vi "Swerve Drive.vi"(0 "X":dbl, 1 "Rot. Point X":dbl, 3 "Rot. Point Y":dbl, 5 "Y":dbl, 7 "Z":dbl, 11 "Error In":errorcluster, 12 "Robot Centric?":bool=TRUE, 13 "Autonomous?":bool, 14 "Yaw":dbl) -> (4 "Front Left Output":dbl, 6 "Front Right Output":dbl, 8 "Back Left Output":dbl, 10 "Back Right Output":dbl, 15 "Error Out":errorcluster)   [LabVIEW 2017]
uses:
  Public/Documents/Cross The Road Electronics/Phoenix-LabVIEW/Motor Controller/Controls/CTRE_Phoenix_MotorControl_ControlMode.ctl
  <vilib>/Rock Robotics/Network Tables/NT Read Number.vi
  <vilib>/Rock Robotics/Network Tables/NT Write Numeric Array.vi
panel:
  in  "Robot Length":dbl=33.5
  in  "Robot Width":dbl=28.5
  # "Swerve Drive Teleoperated Control\nFRC Team 34"
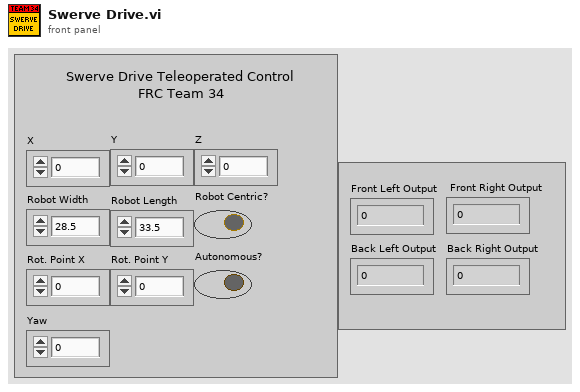
[diagram p1: front panel]
types:
  T1 = enum16{"Front Left", "Front Right", "Back Left", "Back Right"}
  T2 = typedef "CTRE_Phoenix_MotorControl_ControlMode.ctl" = u16
  T3 = typedef "WPI_MotorControlDeviceRef.ctl" = cluster{"DeviceStatus":errorcluster, "Type":T4, "PWM":cluster{"PWM Channel":T5, "DeadBand":T6}, "CAN":cluster{"Device Number":u8, "SetOutput VI Ref":variant, "GetOutput VI Ref":variant, "Enable VI Ref":variant, "Disable VI Ref":variant, "Data":variant}, "Invert":bool, "DIO PWM":cluster{"PWM \"Enable\" Channel":T5, "DIOChannel":T7, "PWM Rate":dbl}}
  T4 = typedef "WPI_MotorControlType.ctl" = enum16{"PWM", "CAN", "DIO PWM"}
  T5 = typedef "FPGA_DIOPWMChannel.ctl" = enum8{"PWM 0", "PWM 1", "PWM 2", "PWM 3", "PWM 4", "PWM 5", "PWM 6", "PWM 7", "PWM 8", "PWM 9", "PWM MXP 0", "PWM MXP 1", "PWM MXP 2", "PWM MXP 3", "PWM MXP 4", "PWM MXP 5", "PWM MXP 6", "PWM MXP 7", "PWM MXP 8", "PWM MXP 9", "Invalid"}
  T6 = typedef "WPI_PWMDeadband.ctl" = cluster{"Name":string, "maxPositivePwm":i32, "minPositivePwm":i32, "centerPwm":i32, "maxNegativePwm":i32, "minNegativePwm":i32, "angularRange":u16}
  T7 = typedef "FPGA_DIOChannel.ctl" = enum8{"DIO 0", "DIO 1", "DIO 2", "DIO 3", "DIO 4", "DIO 5", "DIO 6", "DIO 7", "DIO 8", "DIO 9", "DIO MXP 0", "DIO MXP 1", "DIO MXP 2", "DIO MXP 3", "DIO MXP 4", "DIO MXP 5", "DIO MXP 6", "DIO MXP 7", "DIO MXP 8", "DIO MXP 9", "DIO MXP 10", "DIO MXP 11", "DIO MXP 12", "DIO MXP 13", "DIO MXP 14", "DIO MXP 15", "SPI Port CS1", "SPI Port CS2", "SPI Port CS3", "SPI Port MISO", "SPI Port MOSI", "Invalid"}
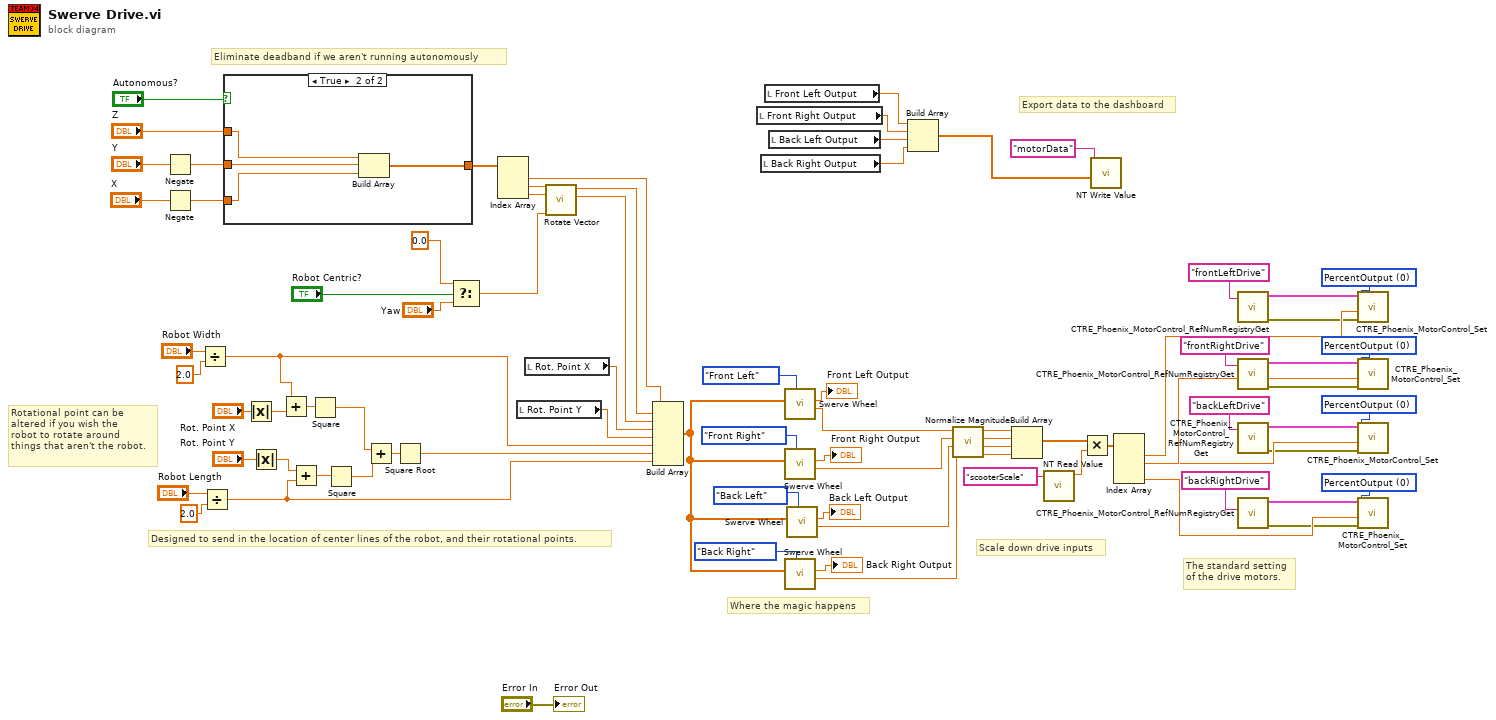
[diagram p0: block diagram]
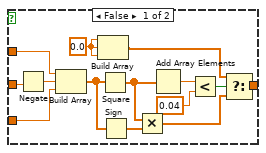
[diagram p2: hidden frame]
diagram:
  w12 = T2 0 items=["PercentOutput"=0, "Position"=1, "Velocity"=2, "Current"=3, "Follower"=5, "MotionProfile"=6, "MotionMagic"=7, "MotionMagicArc"=8, "MotionProfileArc"=10, "Disabled"=15] ("Control Mode")
  w13 = T2 0 items=["PercentOutput"=0, "Position"=1, "Velocity"=2, "Current"=3, "Follower"=5, "MotionProfile"=6, "MotionMagic"=7, "MotionMagicArc"=8, "MotionProfileArc"=10, "Disabled"=15] ("Control Mode")
  w14 = T2 0 items=["PercentOutput"=0, "Position"=1, "Velocity"=2, "Current"=3, "Follower"=5, "MotionProfile"=6, "MotionMagic"=7, "MotionMagicArc"=8, "MotionProfileArc"=10, "Disabled"=15] ("Control Mode")
  w15 = T2 0 items=["PercentOutput"=0, "Position"=1, "Velocity"=2, "Current"=3, "Follower"=5, "MotionProfile"=6, "MotionMagic"=7, "MotionMagicArc"=8, "MotionProfileArc"=10, "Disabled"=15] ("Control Mode")
  # "Export data to the dashboard"
  # "Rotational point can be \naltered if you wish the \nrobot to rotate around \nthings that aren't the robot."
  # "Scale down drive inputs"
  # "Eliminate deadband if we aren't running autonomously"
  # "Where the magic happens"
  # "The standard setting\nof the drive motors."
  # "Designed to send in the location of center lines of the robot, and their rotational points."
  n1 = Negate(x="Y") -> (-x=w33:dbl)
  n2 = Negate(x="X") -> (-x=w32:dbl)
  n3 = Divide(x="Robot Width", y=2.0) -> (x/y=w55:dbl)
  n4 = Divide(x="Robot Length", y=2.0) -> (x/y=w53:dbl)
  n5 = case shown="True" "Autonomous?" {
    tunnel: w33 -> [w86 w99]
    tunnel: [w85 w97] -> w81
    tunnel: "Z" -> [w84 w100]
    tunnel: w32 -> [w83 w98]
    frame False {
      w92 = 0.0 ("element")
      n6 = Negate(x=w86) -> (-x=w88:dbl)
      n7 = Build Array(w84, w88, w83) -> (w91:dbl[])
      n8 = Build Array(w92, w92, w92) -> (w93:dbl[])
      n9 = Square(x=w91) -> (x^2=w89:dbl[])
      n10 = Sign(1:w91) -> (0:w90:dbl[])
      n11 = Multiply(x=w89, y=w90) -> (x*y=w87:dbl[])
      n12 = Add Array Elements(numeric array=w89) -> (sum=w96:dbl)
      n13 = Less?(x=w96, y=0.04 ("x")) -> (x < y?=w94:bool)
      n14 = Select(t=w93, s=w94, f=w87) -> (s? t:f=w85:dbl[])
    }
    frame True {
      n15 = Build Array(w100, w99, w98) -> (w97:dbl[])
    }
  }
  n16 = Absolute Value(x="Rot. Point X") -> (abs(x)=w67:dbl)
  n17 = Absolute Value(x="Rot. Point Y") -> (abs(x)=w64:dbl)
  n18 = Add(x=w55, y=w67) -> (x+y=w66:dbl)
  n19 = Add(x=w64, y=w53) -> (x+y=w65:dbl)
  n20 = Square(x=w66) -> (x^2=w62:dbl)
  n21 = Square(x=w65) -> (x^2=w63:dbl)
  n22 = Add(x=w62, y=w63) -> (x+y=w61:dbl)
  n23 = Square Root(x=w61) -> (sqrt(x)=w54:dbl)
  n24 = Select(t=0.0, s="Robot Centric?", f="Yaw") -> (s? t:f=w74:dbl)
  n25 = Index Array(array=w81) -> (element #1=w60:dbl, element #2=w76:dbl, element #3=w75:dbl)  [unwired: 3 in]
  n26 = local read "Rot. Point Y"() -> (w56:dbl)
  n27 = local read "Rot. Point X"() -> (w57:dbl)
  n28 = call "Rotate Vector.vi"("Angle"=w74, "X"=w75, "Y"=w76) -> ("X'"=w58:dbl, "Y'"=w59:dbl)  [unwired: 7 in]
  n29 = Build Array(w60, w59, w58, w57, w56, w55, w54, w53) -> (w52:dbl[])
  n30 = local read "Front Right Output"() -> (w8:dbl)
  n31 = local read "Back Right Output"() -> (w6:dbl)
  n32 = local read "Front Left Output"() -> (w9:dbl)
  n33 = local read "Back Left Output"() -> (w7:dbl)
  n34 = call "Swerve Wheel.vi"("Wheel"=T1."Front Left", "Inputs"=w52) -> ("Speed"=w49:dbl, "Motor Output"=→"Front Left Output":dbl)  [unwired: 8 in]
  n35 = call "Swerve Wheel.vi"("Wheel"=T1."Front Right", "Inputs"=w52) -> ("Speed"=w48:dbl, "Motor Output"=→"Front Right Output":dbl)  [unwired: 8 in]
  n36 = call "Swerve Wheel.vi"("Wheel"=T1."Back Right", "Inputs"=w52) -> ("Speed"=w46:dbl, "Motor Output"=→"Back Right Output":dbl)  [unwired: 8 in]
  n37 = call "Swerve Wheel.vi"("Wheel"=T1."Back Left", "Inputs"=w52) -> ("Speed"=w47:dbl, "Motor Output"=→"Back Left Output":dbl)  [unwired: 8 in]
  n38 = Build Array(w9, w8, w7, w6) -> (w11:dbl[])
  n39 = call "Normalize Magnitude.vi"("D"=w46, "C"=w47, "B"=w48, "A"=w49) -> ("D'"=w42:dbl, "C'"=w43:dbl, "B'"=w44:dbl, "A'"=w45:dbl)  [unwired: 4 in]
  n40 = Build Array(w45, w44, w43, w42) -> (w41:dbl[])
  n41 = call-poly <vilib>:"NT Read Value.vi"("Name"="scooterScale") -> ("Numeric"=w39:dbl)  [unwired: 9 in, 1 out]
  n42 = Multiply(x=w41, y=w39) -> (x*y=w38:dbl[])
  n43 = call-poly <vilib>:"NT Write Value.vi"("Numeric Array"=w11, "Name"="motorData") -> ()  [unwired: 9 in, 1 out]
  n44 = Index Array(array=w38) -> (element #1=w26:dbl, element #2=w20:dbl, element #3=w17:dbl, element #4=w23:dbl)  [unwired: 4 in]
  n45 = call "CTRE_Phoenix_MotorControl_RefNumRegistryGet.vi"("refnum name"="frontLeftDrive") -> ("error out"=w25:errorcluster, "PhoenixMotorControlDevRef"=w27:T3)  [unwired: 9 in]
  n46 = call "CTRE_Phoenix_MotorControl_RefNumRegistryGet.vi"("refnum name"="frontRightDrive") -> ("error out"=w19:errorcluster, "PhoenixMotorControlDevRef"=w21:T3)  [unwired: 9 in]
  n47 = call "CTRE_Phoenix_MotorControl_RefNumRegistryGet.vi"("refnum name"="backLeftDrive") -> ("error out"=w16:errorcluster, "PhoenixMotorControlDevRef"=w18:T3)  [unwired: 9 in]
  n48 = call "CTRE_Phoenix_MotorControl_RefNumRegistryGet.vi"("refnum name"="backRightDrive") -> ("error out"=w22:errorcluster, "PhoenixMotorControlDevRef"=w24:T3)  [unwired: 9 in]
  n49 = call "CTRE_Phoenix_MotorControl_Set.vi"("error in (no error)"=w25, "Output"=w26, "Control Mode"=w15, "PhoenixMotorControlDevRef"=w27) -> ()  [unwired: 6 in, 2 out]
  n50 = call "CTRE_Phoenix_MotorControl_Set.vi"("error in (no error)"=w19, "Output"=w20, "Control Mode"=w14, "PhoenixMotorControlDevRef"=w21) -> ()  [unwired: 6 in, 2 out]
  n51 = call "CTRE_Phoenix_MotorControl_Set.vi"("error in (no error)"=w16, "Output"=w17, "Control Mode"=w13, "PhoenixMotorControlDevRef"=w18) -> ()  [unwired: 6 in, 2 out]
  n52 = call "CTRE_Phoenix_MotorControl_Set.vi"("error in (no error)"=w22, "Output"=w23, "Control Mode"=w12, "PhoenixMotorControlDevRef"=w24) -> ()  [unwired: 6 in, 2 out]
  "Error Out" <- "Error In"
